vi "Keithley 6517 Perform Zero Correction.vi"() -> ()   [LabVIEW 2016]
doc: "This example shows how to perform zero correction.\n\n<B>Note:</B>\nThis Example is compatible with both model 6517 and 6514."
uses:
  <instrlib>/Keithley 6517/Keithley 6517.lvlib
panel:
  in  "Instrument Model":i32(ring) items=["MODEL 6517B", "MODEL 6517A", "MODEL 6514"]
  out "Measurement":T1 {"Measurement" format="%.6e"}
  in  "VISA resource name":refnum<visa-resource-name>
  # "(c) 2016-2017 National Instruments.  ALL RIGHTS RESERVED."
  # "Note: This Example is compatible with model 6517 and 6514."
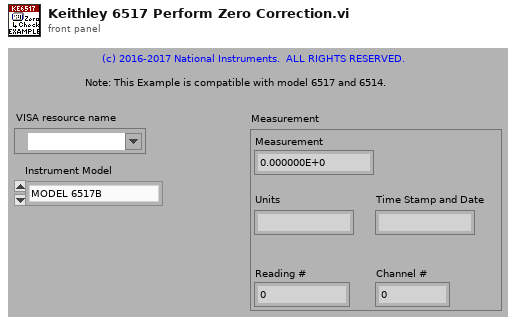
[diagram p1: front panel]
types:
  T1 = cluster{"Measurement":dbl, "Units":string, "Time Stamp and Date":string, "Reading #":dbl, "Channel #":dbl}
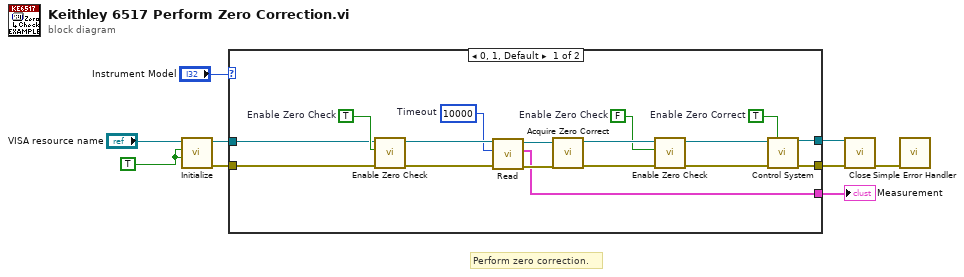
[diagram p0: block diagram]
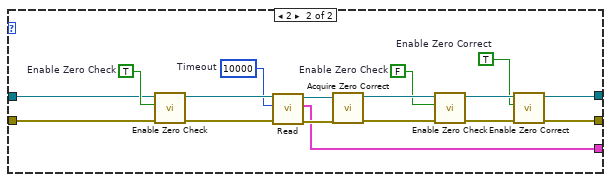
[diagram p2: hidden frame]
diagram:
  w3 = TRUE ("ID Query (True)")
  # "Perform zero correction."
  n1 = call <instrlib>:"Initialize.vi"("Reset (True)"=w3, "ID Query (True)"=w3, "VISA resource name"="VISA resource name") -> ("error out"=w7:errorcluster, "VISA resource name out"=w8:refnum<visa-resource-name>)  [unwired: 7 in]
  n2 = case shown="0, 1, Default" "Instrument Model" {
    tunnel: w8 -> [w19 w39]
    tunnel: w7 -> [w18 w38]
    tunnel: [w17 w29] -> w5
    tunnel: [w16 w30] -> w4
    tunnel: [w10 w32] -> w2
    frame 0, 1, Default {
      w11 = u32 10000  # Timeout
      w22 = FALSE  # Enable Zero Check
      w25 = TRUE  # Enable Zero Correct
      w26 = TRUE  # Enable Zero Check
      n3 = call <instrlib>:"Enable Zero Check.vi"("error in (no error)"=w18, "Enable Zero Check (T: Enable)"=w26, "VISA resource name"=w19) -> ("error out"=w12:errorcluster, "VISA resource name out"=w13:refnum<visa-resource-name>)  [unwired: 7 in]
      n4 = call <instrlib>:"Read.vi"("error in (no error)"=w12, "Timeout(10000 ms)"=w11, "VISA resource name"=w13) -> ("error out"=w15:errorcluster, "Measurement"=w10:T1, "VISA resource name out"=w14:refnum<visa-resource-name>)  [unwired: 6 in]
      n5 = call <instrlib>:"Acquire Zero Correct.vi"("error in (no error)"=w15, "VISA resource name"=w14) -> ("error out"=w23:errorcluster, "VISA resource name out"=w24:refnum<visa-resource-name>)  [unwired: 8 in]
      n6 = call <instrlib>:"Enable Zero Check.vi"("error in (no error)"=w23, "Enable Zero Check (T: Enable)"=w22, "VISA resource name"=w24) -> ("error out"=w20:errorcluster, "VISA resource name out"=w21:refnum<visa-resource-name>)  [unwired: 7 in]
      n7 = call <instrlib>:"Control System.vi"("VISA resource name"=w21, "Enable Zero Correct (F: Disable)"=w25, "error in (no error)"=w20) -> ("VISA resource name out"=w17:refnum<visa-resource-name>, "error out"=w16:errorcluster)  [unwired: 11 in]
    }
    frame 2 {
      w27 = TRUE  # Enable Zero Correct
      w33 = u32 10000  # Timeout
      w40 = FALSE  # Enable Zero Check
      w43 = TRUE  # Enable Zero Check
      n8 = call <instrlib>:"Enable Zero Check.vi"("error in (no error)"=w38, "Enable Zero Check (T: Enable)"=w43, "VISA resource name"=w39) -> ("error out"=w34:errorcluster, "VISA resource name out"=w35:refnum<visa-resource-name>)  [unwired: 7 in]
      n9 = call <instrlib>:"Read.vi"("error in (no error)"=w34, "Timeout(10000 ms)"=w33, "VISA resource name"=w35) -> ("error out"=w37:errorcluster, "Measurement"=w32:T1, "VISA resource name out"=w36:refnum<visa-resource-name>)  [unwired: 6 in]
      n10 = call <instrlib>:"Acquire Zero Correct.vi"("error in (no error)"=w37, "VISA resource name"=w36) -> ("error out"=w41:errorcluster, "VISA resource name out"=w42:refnum<visa-resource-name>)  [unwired: 8 in]
      n11 = call <instrlib>:"Enable Zero Check.vi"("error in (no error)"=w41, "Enable Zero Check (T: Enable)"=w40, "VISA resource name"=w42) -> ("error out"=w31:errorcluster, "VISA resource name out"=w28:refnum<visa-resource-name>)  [unwired: 7 in]
      n12 = call <instrlib>:"Enable Zero Correct.vi"("error in (no error)"=w31, "Enable Zero Correct (F: Disable)"=w27, "VISA resource name"=w28) -> ("error out"=w30:errorcluster, "VISA resource name out"=w29:refnum<visa-resource-name>)  [unwired: 7 in]
    }
  }
  "Measurement" <- w2
  n13 = call <instrlib>:"Close.vi"("error in (no error)"=w4, "VISA resource name"=w5) -> ("error out"=w6:errorcluster)  [unwired: 9 in]
  n14 = call <vilib>:"Simple Error Handler.vi"("error in (no error)"=w6) -> ()  [unwired: 4 in, 5 out]
